vi "Read Water Level Actor.vi"(11 "HW Evaporative Cooler":refnum<class "HW Evaporative Cooler.lvclass">) -> (2 "Water Level":refnum<class "Water Level.lvclass">)   [LabVIEW 2025, in "HW Evaporative Cooler.lvclass"]
uses:
  HW Evaporative Cooler.lvclass
  Water Level/Water Level.lvclass
  HW Water Level.lvclass/HW Water Level.lvclass
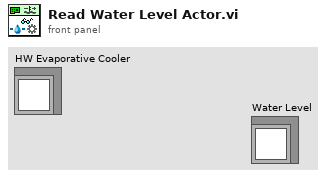
[diagram p1: front panel]
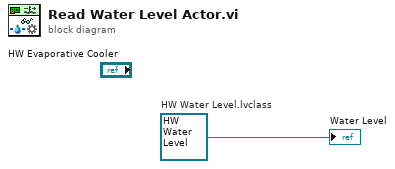
[diagram p0: block diagram]
diagram:
  w1 = refnum<class "HW Water Level.lvclass"> refnum  # HW Water Level.lvclass
  "Water Level" <- w1
